vi "GV_SubScribe_to_server.vi"(8 "error in (no error)":errorcluster, 10 "Gviewer-name":string, 11 "Gviewer in":refnum<class "Gviewer.lvclass">) -> (0 "error out":errorcluster, 3 "Gviewer out":refnum<class "Gviewer.lvclass">)   [LabVIEW 2020, in "Sgraph_lib_V1.lvlib" / "Gviewer.lvclass"]
doc: "Subscribe to the Gserver Queue or Network"
uses:
  Gviewer.lvclass
  Gviewer.lvclass/Gviewer.ctl
  Gserver/controls/Typedef_Gviewer-Query.ctl
  Gserver/controls/Typedef_QueryType.ctl
  controls/Typedef_Gserver-Replies.ctl
  controls/Typedef_ServerActions.ctl
  Gserver/Gserver.lvclass
  Builds/Sgraph_lib_V1.lvlib
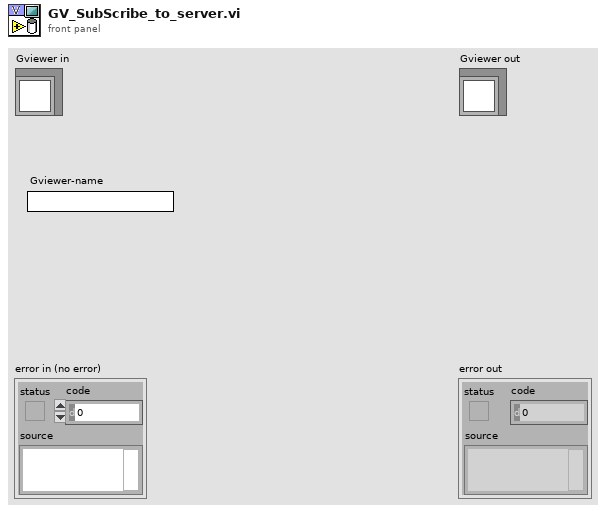
[diagram p1: front panel]
types:
  T1 = typedef "Typedef_Gserver-Replies.ctl" = cluster{"ServerActions":T2, "data":variant, "Source":string, "Time Stamp":timestamp}
  T2 = typedef "Sgraph_lib_V1.lvlib/Gviewer.lvclass/Typedef_ServerActions.ctl" = enum16{"GraphUpdate", "SendAllTags", "SendIniPath", "SetGeneralOptions", "EditTagsOpen", "EditTagsPresetSave", "EditTagsPresetLoad", "EditTagsClose", "NewTagSelection", "AutoScale", "DBeditStatus", "DBsaveConfirm", "GetXconstraints", "ExitGraph"}
  T3 = typedef "Sgraph_lib_V1.lvlib/Gserver.lvclass/Typedef_QueryType.ctl" = enum16{"Subscribe", "SubscribeNetw", "DataRequest", "RequestAllTags", "RequestIniPath", "FAMMstarted", "SetClientOptions", "GviewerUpdate", "OpenNewGraph", "CloseClient", "CloseAllClients", "Close Gserver", "OpenMemoryMap", "MeMapDataRequest", "MeMapDataResponse", "OpenDBeditor", "CheckDBeditorRunning", "StoppedDBeditor", "SaveDB_TAGpropRecord", "ConfirmDB_TAGpropSave", "GetXconstraints", "OpenNewNetworkGraph"}
  T4 = typedef "Sgraph_lib_V1.lvlib/Gserver.lvclass/Typedef_Gviewer-Query.ctl" = cluster{"Query_type":T3, "data":variant, "Source":string, "Time Stamp":timestamp}
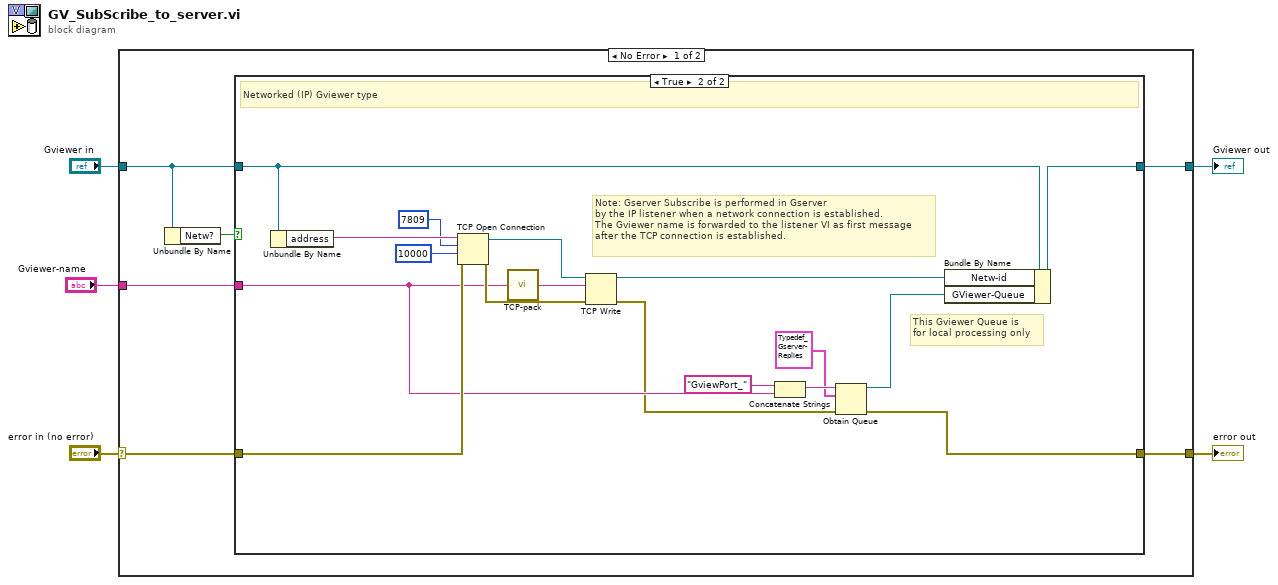
[diagram p0: block diagram]
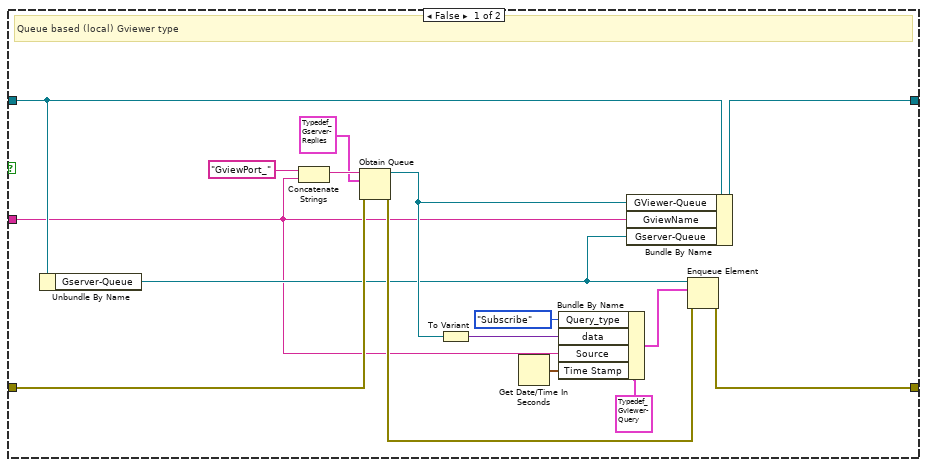
[diagram p2: hidden frame]
diagram:
  n1 = case shown="No Error" "error in (no error)" {
    selector: "error in (no error)" -> [w9 w46]
    tunnel: [w8 w46] -> w4
    tunnel: [w7 w45] -> w2
    tunnel: "Gviewer in" -> [w10 w45]
    tunnel: "Gviewer-name" -> [w6 _]
    frame No Error {
      n2 = Unbundle By Name(w10) -> ("Netw?"=w11:bool)
      n3 = case shown="True" w11 {
        tunnel: w10 -> [w14 w39]
        tunnel: w9 -> [w16 w43]
        tunnel: [w15 w29] -> w8
        tunnel: [w17 w40] -> w7
        tunnel: w6 -> [w12 w31]
        frame False {
          # "Queue based (local) Gviewer type"
          n4 = Unbundle By Name(w14) -> ("Gserver-Queue"=w13:refnum<queue>)
          n5 = Concatenate Strings("GviewPort_", w12) -> (w22:string)
          n6 = Obtain Queue(name (unnamed)=w22, element data type=T1 {"ServerActions"=enum."GraphUpdate", "data"=variant, "Source"="", "Time Stamp"=timestamp(0 s since 1904-01-01)} ("Query"), error in (no error)=w16) -> (queue out=w18:refnum<queue>, error out=w21:errorcluster)  [unwired: 2 in, 1 out]
          n7 = To Variant(anything=w18) -> (Variant=w19:variant)
          n8 = Get Date/Time In Seconds() -> (seconds since 1Jan1904=w24:timestamp)
          n9 = Bundle By Name(cluster=T4 {"Query_type"=enum."Subscribe", "data"=variant, "Source"="", "Time Stamp"=timestamp(0 s since 1904-01-01)} ("element"), "Query_type"=Typedef_QueryType."Subscribe", "data"=w19, "Source"=w12, "Time Stamp"=w24) -> (w26:T4)
          n10 = Bundle By Name(cluster=w14, "GViewer-Queue"=w18, "GviewName"=w12, "Gserver-Queue"=w13) -> (w17:refnum<class "Gviewer.lvclass">)
          n11 = Enqueue Element(queue=w13, element=w26, error in (no error)=w21) -> (error out=w15:errorcluster)  [unwired: 1 in, 2 out]
        }
        frame True {
          # "This Gviewer Queue is\nfor local processing only"
          # "Note: Gserver Subscribe is performed in Gserver\nby the IP listener when a network connection is established.\nThe Gviewer name is forwarded to the listener VI as first message\nafter the TCP connection is established."
          # "Networked (IP) Gviewer type"
          n12 = Unbundle By Name(w39) -> ("address"=w44:string)
          n13 = TCP Open Connection(address=w44, remote port or service name=u16 7809, timeout ms (60000)=10000, error in (no error)=w43) -> (connection ID=w37:refnum<k5>, error out=w35:errorcluster)  [unwired: 1 in]
          n14 = call "TCP-pack.vi"("Data to send"=w31) -> ("Data toTCP"=w38:string)  [unwired: 6 in]
          n15 = TCP Write(connection ID=w37, data in=w38, error in (no error)=w35) -> (connection ID out=w36:refnum<k5>, error out=w30:errorcluster)  [unwired: 1 in, 1 out]
          n16 = Concatenate Strings("GviewPort_", w31) -> (w33:string)
          n17 = Obtain Queue(name (unnamed)=w33, element data type=T1 {"ServerActions"=enum."GraphUpdate", "data"=variant, "Source"="", "Time Stamp"=timestamp(0 s since 1904-01-01)} ("Query"), error in (no error)=w30) -> (queue out=w28:refnum<queue>, error out=w29:errorcluster)  [unwired: 2 in, 1 out]
          n18 = Bundle By Name(cluster=w39, "Netw-id"=w36, "GViewer-Queue"=w28) -> (w40:refnum<class "Gviewer.lvclass">)
        }
      }
    }
    frame Error {
    }
  }
  "error out" <- w4
  "Gviewer out" <- w2
